vi "Set Groups.vi"(8 "error in (no error)":errorcluster, 10 "Groups":refnum<class "Group.lvclass">[](array[class]), 11 "DataLogger in":refnum<class "DataLogger.lvclass">) -> (0 "error out":errorcluster, 3 "DataLogger out":refnum<class "DataLogger.lvclass">)   [LabVIEW 2020, in "VolatusData.lvlib" / "DataLogger.lvclass"]
uses:
  DataLogger.lvclass
  lv-vecto/Vecto/Group/Group.lvclass
  DataLogger.lvclass/DataLogger.ctl
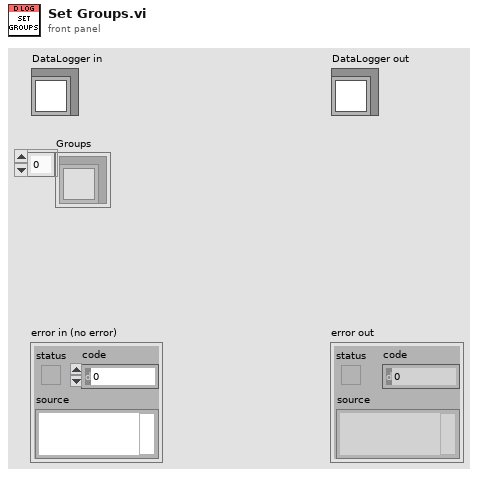
[diagram p1: front panel]
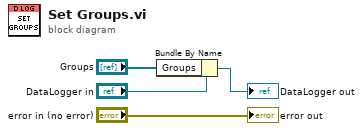
[diagram p0: block diagram]
diagram:
  n1 = Bundle By Name(cluster="DataLogger in", "Groups"="Groups") -> (→"DataLogger out":refnum<class "DataLogger.lvclass">)
  "error out" <- "error in (no error)"
